vi "rpm manuale global.vi"() -> ()   [LabVIEW 2019]
panel:
  out "rpm manuale":dbl
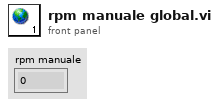
[diagram p1: front panel]
diagram:
